vi "ma_SML Moving Average Linear Weighting.vi"(0 "x(n)":dbl[](array[numeric]) format="%.2f", 1 "y(n-1)":dbl[](array[numeric]) format="%.2f", 2 "averaged sofar(n-1)":dbl format="%.2f", 3 "average size":dbl format="%.2f", 4 "reset?":bool) -> (5 "y(n)":dbl[](array[numeric]) format="%.2f", 6 "averaged sofar(n)":dbl format="%.2f")   [LabVIEW 2020, in "NI_MAPro.lvlib"]
uses:
  NI_MAPro.lvlib
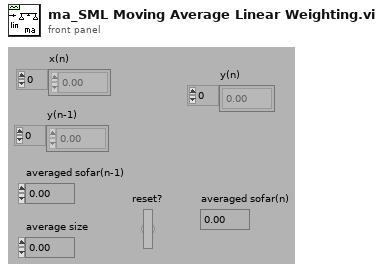
[diagram p1: front panel]
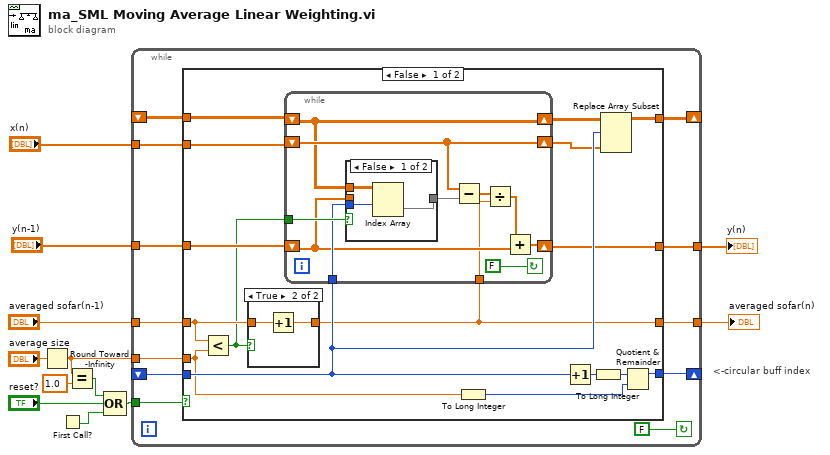
[diagram p0: block diagram]
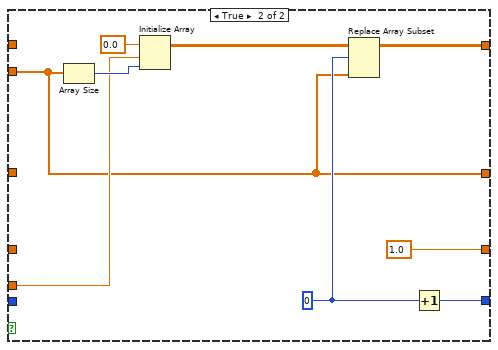
[diagram p4: hidden frame]
diagram:
  # "<-circular buff index"
  n1 = Round Toward -Infinity(1:"average size") -> (0:w2:dbl)
  n2 = First Call?() -> (First Call?: T/F=w4:bool)
  n3 = Equal?(x=w2, y=1.0) -> (x = y?=w3:bool)
  n4 = Compound Arithmetic op=OR(w3, "reset?", w4) -> (w5:bool)
  n5 = while {
    tunnel: [w14] -> w7
    tunnel: "averaged sofar(n-1)" -> [w15]
    tunnel: [w16] -> w6
    tunnel: "y(n-1)" -> [w17]
    tunnel: w2 -> [w21]
    tunnel: "x(n)" -> [w22]
    shift-left: _ -> [w19]
    shift-right: [w23] -> _
    shift-left: _ -> [w18]
    shift-right: [w20] -> _
    tunnel: w5 -> [w24]
    stop <- FALSE continue-if-true
    n6 = case shown="False" w24 {
      tunnel: [w40 w64] -> w23
      tunnel: w22 -> [w36 w59]
      tunnel: w21 -> [w31 w61]
      tunnel: [w33 w63] -> w20
      tunnel: [w30 1.0] -> w14
      tunnel: [w32 w59] -> w16
      tunnel: w19 -> [w34 _]
      tunnel: w15 -> [w29 _]
      tunnel: w17 -> [w35 _]
      tunnel: w18 -> [w37 _]
      frame False {
        n7 = Less?(x=w29, y=w31) -> (x < y?=w28:bool)
        n8 = case shown="True" w28 {
          tunnel: w29 -> [w56 w58]
          tunnel: [w56 w57] -> w30
          frame False {
          }
          frame True {
            n9 = Increment(x=w58) -> (x+1=w57:dbl)
          }
        }
        n10 = while {
          tunnel: w28 -> [w50]
          tunnel: w30 -> [w42]
          shift-left: w36 -> [w51]
          shift-right: [w51] -> w26
          shift-left: w35 -> [w46]
          shift-right: [w45] -> w32
          tunnel: w34 -> [w48]
          shift-left: w37 -> [w47]
          shift-right: [w47] -> w27
          stop <- FALSE continue-if-true
          n11 = case shown="False" w50 {
            tunnel: [w52 w55] -> w49
            tunnel: w46 -> [_ w55]
            tunnel: w48 -> [w54 _]
            tunnel: w47 -> [w53 _]
            frame False {
              n12 = Index Array(array=w53, index (row)=w54) -> (element=w52:dbl[])  [unwired: 1 in]
            }
            frame True {
            }
          }
          n13 = Subtract(x=w51, y=w49) -> (x-y=w43:dbl[])
          n14 = Divide(x=w43, y=w42) -> (x/y=w44:dbl[])
          n15 = Add(x=w44, y=w46) -> (x+y=w45:dbl[])
        }
        n16 = To Long Integer(number=w31) -> (32bit integer=w25:i32)
        n17 = Increment(x=w34) -> (x+1=w39:i32)
        n18 = To Long Integer(number=w39) -> (32bit integer=w38:i32)
        n19 = Replace Array Subset(array=w27, new element=w26, index (row)=w34) -> (w33:dbl[][])  [unwired: 1 in]
        n20 = Quotient & Remainder(x=w38, y=w25) -> (x-y*floor(x/y)=w40:i32)  [unwired: 1 out]
      }
      frame True {
        w62 = 0
        n21 = Array Size(array=w59) -> (size(s)=w67:i32)
        n22 = Initialize Array(0.0 ("Element Data"), w61, w67) -> (w60:dbl[][])
        n23 = Replace Array Subset(array=w60, new element=w59, index (row)=w62) -> (w63:dbl[][])  [unwired: 1 in]
        n24 = Increment(x=w62) -> (x+1=w64:i32)
      }
    }
  }
  "averaged sofar(n)" <- w7
  "y(n)" <- w6
